vi "set design tool filepaths.vi"(8 "error in (no error)":errorcluster) -> (0 "error out":errorcluster, 1 "Completed Designs":path, 2 "Requested Designs":path, 3 "Design Tool":path, 4 "Methods":string[](array[string]), 6 "Success":bool)   [LabVIEW 2011, in "Design Server.lvlib"]
uses:
  Design Server.lvlib
  Folders.ctl
  <vilib>/Utility/config.llb/Read Key (Path).vi
  Instance           3 33Saved   set design tool filepaths .vi
  <vilib>/Utility/config.llb/Write Key (Path).vi
  <vilib>/Utility/config.llb/NI_LVConfig.lvlib
panel:
  out "File Paths":path[](array[path])
  out "application name":string
  out "Prompt":string[](array[string])
  out "Key":string[](array[string])
  in  "Folders":T1
  # "3 folders\nFInal Designs\nFolder with incoming requests\nFolder with completed designs"
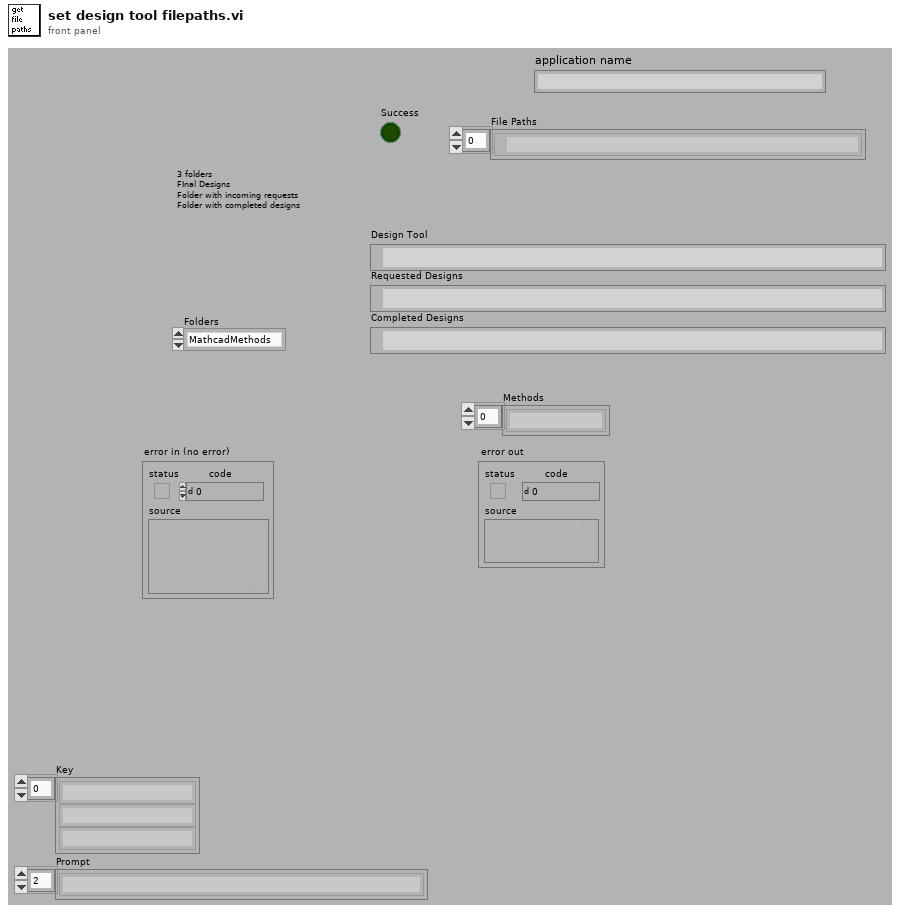
[diagram p1: front panel]
types:
  T1 = typedef "Design Server.lvlib/Folders.ctl" = enum16{"MathcadMethods", "RequestedDesigns", "CompletedDesigns", "MathcadCode", "CollabnetSVN.exe"}
  T2 = typedef "NI_LVConfig.lvlib/Config Data RefNum.ctl" = refnum<k1>
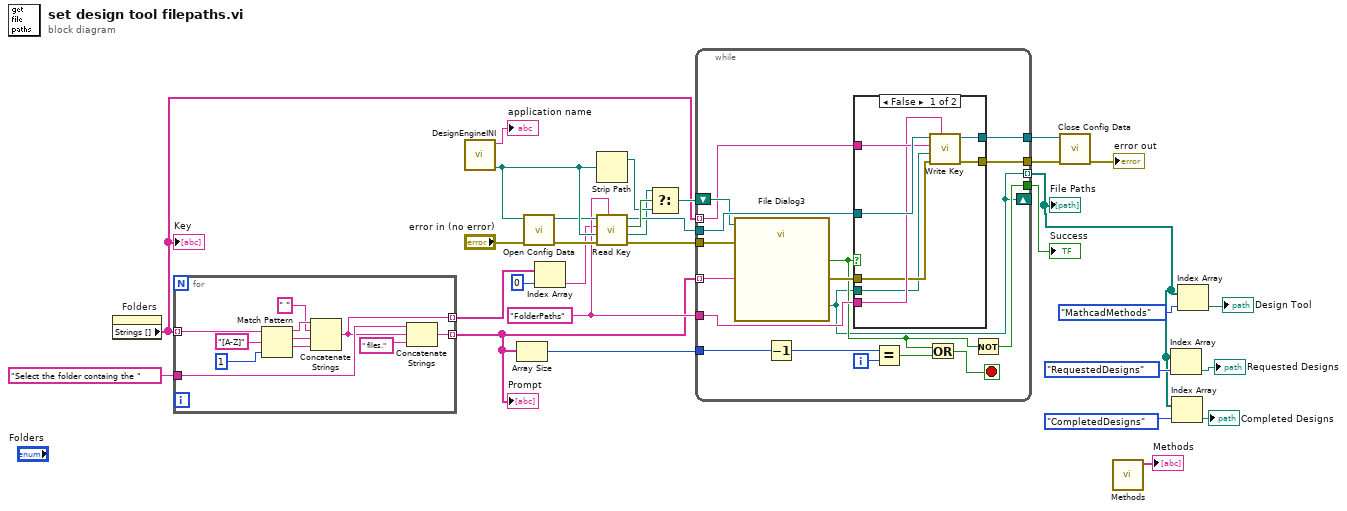
[diagram p0: block diagram]
diagram:
  w16 = "FolderPaths" ("section")
  n1 = property on="Folders" class="Enum (strict)"() -> ("Strings []"=w9:string[])  [unwired: 2 in, 2 out]
  "Key" <- w9
  n2 = for {
    tunnel: w9 -> [w42] mode=indexing
    tunnel: [w32] -> w13 mode=indexing
    tunnel: "Select the folder containg the " -> [w35]
    tunnel: [w33] -> w14 mode=indexing
    n3 = Match Pattern(string=w42, regular expression="[A-Z]", offset (0)=1) -> (before substring=w40:string, match substring=w39:string, after substring=w38:string)  [unwired: 1 out]
    n4 = Concatenate Strings(w40, " " ("string"), w39, w38) -> (w32:string)
    n5 = Concatenate Strings(w35, w32, " files." ("string")) -> (w33:string)
  }
  "Prompt" <- w14
  n6 = call "DesignEngineINI.vi"() -> ("Ini file path"=w30:path, "Application Name"=→"application name":string)  [unwired: 6 in]
  n7 = Array Size(array=w14) -> (size(s)=w18:i32)
  n8 = call <vilib>:"Open Config Data.vi"("error in (no error)"="error in (no error)", "configuration file path"=w30) -> ("error out"=w28:errorcluster, "refnum"=w29:T2)  [unwired: 7 in, 1 out]
  n9 = Index Array(array=w13, index=0) -> (element=w11:string)
  n10 = Strip Path(path=w30) -> (stripped path=w21:path)  [unwired: 1 out]
  n11 = call-poly <vilib>:"Read Key.vi"("section"=w16, "error in (no error)"=w28, "default value"=w30, "key"=w11, "refnum"=w29) -> ("error out"=w25:errorcluster, "value"=w20:path, "found?"=w31:bool, "refnum out"=w26:T2)  [unwired: 3 in]
  n12 = Select(t=w20, s=w31, f=w21) -> (s? t:f=w19:path)
  n13 = while {
    tunnel: w14 -> [w45] mode=indexing
    shift-right: [w43] -> _
    shift-left: w19 -> [w53]
    tunnel: w26 -> [w59]
    tunnel: w16 -> [w58]
    tunnel: w25 -> [w56]
    tunnel: [w55] -> w23
    tunnel: [w54] -> w22
    tunnel: w18 -> [w51]
    tunnel: [w46] -> w17
    tunnel: w9 -> [w44] mode=indexing
    tunnel: [w43] -> w5 mode=indexing
    i -> [w49]
    stop <- w52 stop-if-true
    n14 = call "File Dialog3"("start path"=w53, "prompt"=w45, "error in"=w56) -> ("selected path"=w43:path, "cancelled"=w47:bool, "error out"=w57:errorcluster)  [unwired: 9 in, 1 out]
    n15 = Decrement(x=w51) -> (x-1=w50:i32)
    n16 = case shown="False" w47 {
      tunnel: w59 -> [w66 w67]
      tunnel: w44 -> [w65 _]
      tunnel: w58 -> [w64 _]
      tunnel: w57 -> [w63 w68]
      tunnel: [w62 w67] -> w55
      tunnel: [w61 w68] -> w54
      tunnel: w43 -> [w60 _]
      frame False {
        n17 = call-poly <vilib>:"Write Key.vi"("section"=w64, "error in (no error)"=w63, "value"=w60, "key"=w65, "refnum"=w66) -> ("error out"=w61:errorcluster, "refnum out"=w62:T2)  [unwired: 4 in, 1 out]
      }
      frame True {
      }
    }
    n18 = Equal?(x=w50, y=w49) -> (x = y?=w48:bool)
    n19 = Or(x=w47, y=w48) -> (x .or. y?=w52:bool)
    n20 = Not(x=w47) -> (.not. x?=w46:bool)
  }
  "Success" <- w17
  "File Paths" <- w5
  n21 = call <vilib>:"Close Config Data.vi"("error in (no error)"=w22, "refnum"=w23) -> ("error out"=→"error out":errorcluster)  [unwired: 8 in, 1 out]
  n22 = call "Methods.vi"() -> ("Methods"=→"Methods":string[])  [unwired: 10 in, 1 out]
  n23 = Index Array(array=w5, index=Folders."RequestedDesigns" ("Folders")) -> (element=→"Requested Designs":path)
  n24 = Index Array(array=w5, index=Folders."CompletedDesigns" ("Folders")) -> (element=→"Completed Designs":path)
  n25 = Index Array(array=w5, index=Folders."MathcadMethods" ("Folders")) -> (element=→"Design Tool":path)
